vi "To IRunnable.vi"(8 "error in":errorcluster, 11 "LabVIEW Object":refnum<class>) -> (0 "error out":errorcluster, 3 "IRunnable":refnum<class "IRunnable.lvclass">)   [LabVIEW 2025]
uses:
  IRunnable.lvclass
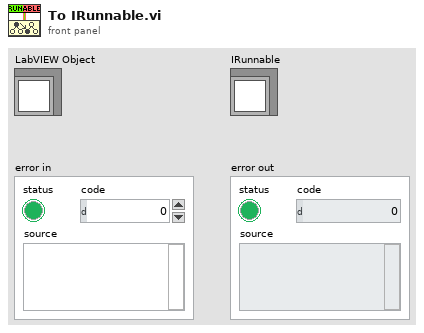
[diagram p1: front panel]
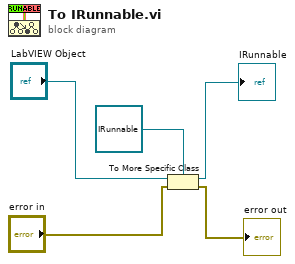
[diagram p0: block diagram]
diagram:
  n1 = To More Specific Class(target class=refnum<class "IRunnable.lvclass"> refnum ("IRunnable.lvclass"), reference="LabVIEW Object", error in="error in") -> (specific class reference=→"IRunnable":refnum<class "IRunnable.lvclass">, error out=→"error out":errorcluster)
